vi "ReadMore.vi"(8 "error in (no error)":errorcluster, 11 "ClientApp1 in":refnum<class "ClientApp1.lvclass">) -> (0 "error out":errorcluster, 2 "Data":string, 3 "ClientApp1 out":refnum<class "ClientApp1.lvclass">)   [LabVIEW 2020, in "ClientApp1Lib.lvlib" / "ClientApp1.lvclass"]
uses:
  ClientApp1.lvclass
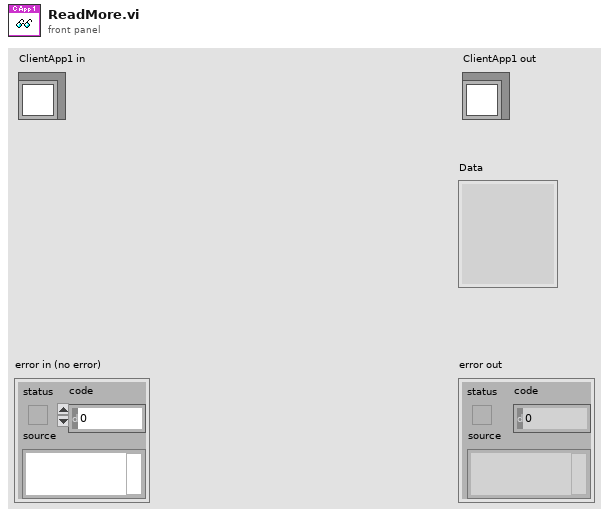
[diagram p1: front panel]
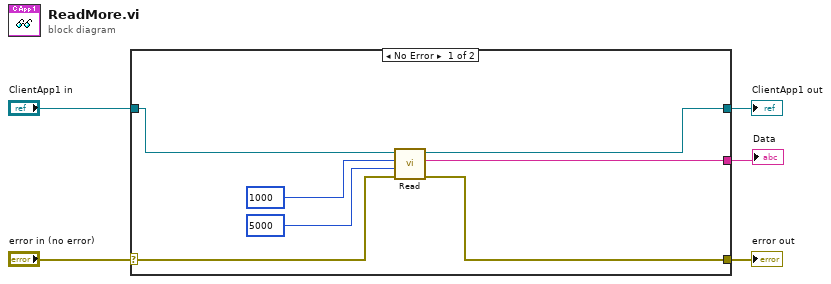
[diagram p0: block diagram]
diagram:
  n1 = case shown="No Error" "error in (no error)" {
    selector: "error in (no error)" -> [w12 w14]
    tunnel: [w11 w14] -> w4
    tunnel: [w7 w13] -> w2
    tunnel: "ClientApp1 in" -> [w6 w13]
    tunnel: [w8 _] -> w1
    frame No Error {
      n2 = call-dynamic "Read.vi"("error in (no error)"=w12, "Timeout"=5000, "NumOfBytes"=1000, "ClientBase in"=w6) -> ("error out"=w11:errorcluster, "Data"=w8:string, "ClientBase out"=w7:refnum<class "ClientApp1.lvclass">)  [unwired: 5 in]
    }
    frame Error {
    }
  }
  "error out" <- w4
  "ClientApp1 out" <- w2
  "Data" <- w1
